vi "String-ReadWrite.vi"(11 "Befehl":string="GAC=123") -> (0 "output 1":u32 format="%8x", 1 "Argument":string, 2 "Befehl,Variable":string, 3 "Enum":enum16{"command", "read", "write"}(ring))   [LabVIEW 2011]
panel:
  out "HexOk":bool
  out "offset past match":i32
  out "match substring":string
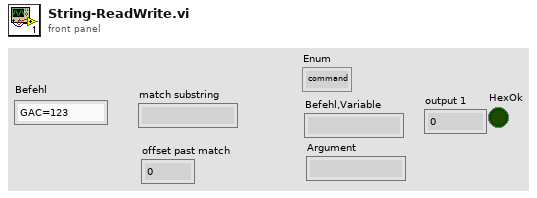
[diagram p1: front panel]
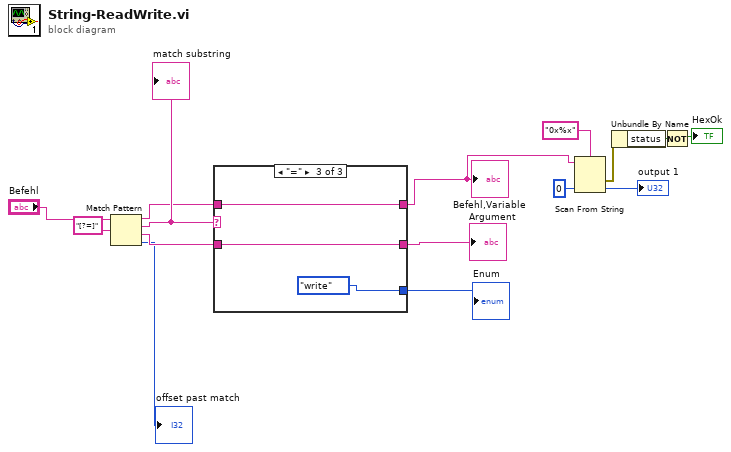
[diagram p0: block diagram]
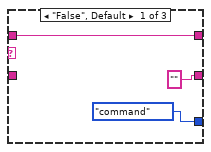
[diagram p2: hidden frame]
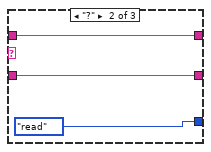
[diagram p3: hidden frame]
diagram:
  n1 = Match Pattern(string="Befehl", regular expression="[?=]") -> (before substring=w11:string, match substring=w13:string, after substring=w12:string, offset past match=→"offset past match":i32)  [unwired: 1 in]
  "match substring" <- w13
  n2 = case shown="\"=\"" w13 {
    tunnel: w12 -> [_ w19 w23]
    tunnel: w11 -> [w17 w21 w24]
    tunnel: [w17 w21 w24] -> w7
    tunnel: ["" ("Befehl") w19 w23] -> w10
    tunnel: [enum16{"command", "read", "write"}."command" ("Enum") enum16{"command", "read", "write"}."read" ("Enum") enum16{"command", "read", "write"}."write" ("Enum")] -> w9
    frame "False", Default {
    }
    frame "?" {
    }
    frame "=" {
    }
  }
  "Argument" <- w10
  "Befehl,Variable" <- w7
  "Enum" <- w9
  n3 = Scan From String(format string="0x%x", input string=w7, default 1=u32 0 ("default value 1")) -> (error out=w4:errorcluster, output 1=→"output 1":u32)  [unwired: 2 in, 2 out]
  n4 = Unbundle By Name(w4) -> ("status"=w3:bool)
  n5 = Not(x=w3) -> (.not. x?=→"HexOk":bool)
